vi "Normliza_AH.vi"(1 "PosAH":dbl) -> (0 "Numeric":dbl)   [LabVIEW 2012]
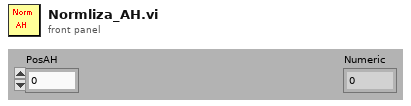
[diagram p1: front panel]
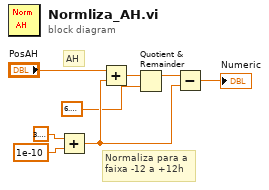
[diagram p0: block diagram]
diagram:
  # "AH"
  # "Normaliza para a\nfaixa -12 a +12h"
  n1 = Add(x=3.141592653589793, y=1e-10) -> (x+y=w4:dbl)
  n2 = Add(x="PosAH", y=w4) -> (x+y=w6:dbl)
  n3 = Quotient & Remainder(x=w6, y=6.283185307179586) -> (x-y*floor(x/y)=w5:dbl)  [unwired: 1 out]
  n4 = Subtract(x=w5, y=w4) -> (x-y=→"Numeric":dbl)
